vi "SVL Unit Conversion.vi"   [LabVIEW 2017]
doc: "Converts between dB/linear, magnitude/magnitude^2, rms/peak/peak-peak, spectrum/spectral density, and dB ref1/dB ref2. You can use this polymorphic VI to convert a single spectrum, N spectra, a single complex spectrum, N complex spectra, a single channel of XY data, N channels of XY data, a single channel with M orders of XY data, N channels with M orders of XY data, waterfall data, or colormap data. The data type you wire to the <B>spectrum</B> or <B>magnitudes</B> input determines the polymorphic instance to use."
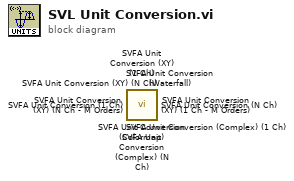
[diagram p0: block diagram]
diagram:
  n1 = call <vilib>:"SVFA Unit Conversion (Colormap).vi"() -> ()  [unwired: 16 in, 4 out]
  n2 = call <vilib>:"SVFA Unit Conversion (Waterfall).vi"() -> ()  [unwired: 16 in, 4 out]
  n3 = call <vilib>:"SVFA Unit Conversion (XY) (N Ch - M Orders).vi"() -> ()  [unwired: 16 in, 4 out]
  n4 = call <vilib>:"SVFA Unit Conversion (XY) (1 Ch - M Orders).vi"() -> ()  [unwired: 16 in, 4 out]
  n5 = call <vilib>:"SVFA Unit Conversion (XY) (N Ch).vi"() -> ()  [unwired: 16 in, 4 out]
  n6 = call <vilib>:"SVFA Unit Conversion (XY) (1 Ch).vi"() -> ()  [unwired: 16 in, 4 out]
  n7 = call <vilib>:"SVFA Unit Conversion (Complex) (N Ch).vi"() -> ()  [unwired: 14 in, 6 out]
  n8 = call <vilib>:"SVFA Unit Conversion (Complex) (1 Ch).vi"() -> ()  [unwired: 14 in, 6 out]
  n9 = call <vilib>:"SVFA Unit Conversion (N Ch).vi"() -> ()  [unwired: 16 in, 4 out]
  n10 = call <vilib>:"SVFA Unit Conversion (1 Ch).vi"() -> ()  [unwired: 16 in, 4 out]
